vi "q2.vi"() -> ()   [LabVIEW 2015]
uses:
  <vilib>/measure/NI_MABase.lvlib
  <vilib>/Analysis/NI_AAL_SigProc.lvlib
panel:
  out "demodulated m2":dbl[](graph)=[0.19117911843553648, 0.5729591319250894, 0.5890890921294468, 1.3154738011707838, 1.3144961866221603, 1.4574064754440013, 1.42216036164409, 1.4832955134231336, 1.3040516378204707, 1.1575885486338888, 0.9909125116259979, 0.7884400558545961, 0.6256179438404917, 0.5043562747351483, 0.37651797922924957, 0.12394215236818269, 0.10483867344378245, 0.1734757640989641, 0.25167677955348666, 0.5258127619495699, 0.6110971369831356, 0.8318077101247057, 0.9128139165643081, 1.1749147514512281, 1.2134698605859797, 1.5175447967871678, 1.4551131185228479, 1.4851009517249243, 1.3185272344601384, 1.1300341180328108, 0.9606799214615833, 0.8187276271950532, 0.6530785676969499, 0.4825772132376491, 0.35900378540456035, 0.1347720355785, 0.11236091609886091, 0.17082168387920313, 0.250995683367065, 0.5240017632339953, 0.6084700995569114, 0.8350791240882549, 0.9160669423121811, 1.172037431329029, 1.2109827917652218, 1.5193252220019504, 1.4564643797442673, 1.4843749689702277, 1.3181101271518103, 1.1300576785179948, 0.9605495874632342, 0.8190225596762173, 0.6534084672462961, 0.48223614388608227, 0.3586916659088199, 0.13502194613968133, 0.11256644243782966, 0.17069219119505608, 0.2509029536063748, 0.5240390189649367, 0.6084824342437518, 0.8350964925844307, 0.9160945289287651, 1.1720012900099623, 1.2109463450464375, 1.5193581407706491, 1.4564930741484268, 1.4843539694936156, 1.3180940037118747, 1.130066624792237, 0.9605549666381606, 0.8190218097926878, 0.6534095504929038, 0.4822330218292607, 0.35868808533895324, 0.13502574918639365, 0.11256999841851738, 0.1706893219238787, 0.2509005340480438, 0.5240406167295595, 0.608483571625249, 0.8350960021102438, 0.9160943330825861, 1.1720011309259701, 1.210946060204705, 1.519358537845759, 1.4564934805140304, 1.4843535931836598, 1.318093672672127, 1.1300668708660897, 0.960555157966931, 0.8190217000510572, 0.6534094821248702, 0.48223303585579635, 0.35868807770087496, 0.13502578178268754, 0.11257003734887348, 0.17068927959896962, 0.2509004934159654, 0.5240406507580907, 0.608483600106657, 0.835095983018602, 0.9160943192608686, 1.1720011372721384, 1.2109460630840572, 1.5193585392010713, 1.4564934834001433, 1.484353588838402, 1.318093668144318, 1.1300668751438718, 0.9605551617662783, 0.8190216971708588, 0.6534094798651788, 0.4822330371897665, 0.3586880785594358, 0.13502578156357317, 0.11257003738314246, 0.170689279262532, 0.25090049299244777, 0.5240406512414064, 0.6084836005711886, 0.8350959826255947, 0.9160943189285427, 1.1720011374994639, 1.2109460632510227, 1.5193585391202487, 1.4564934833598324, 1.4843535888283999, 1.3180936681155528, 1.1300668751910647, 0.9605551618163553, 0.8190216971223002, 0.6534094798217547, 0.4822330372233053, 0.3586880785860207, 0.13502578154758946, 0.11257003737242735, 0.1706892792657163, 0.25090049299265743, 0.5240406512448724, 0.6084836005757819, 0.8350959826202083, 0.9160943189232835, 1.1720011375039954, 1.2109460632548807, 1.5193585391175606, 1.4564934833578214, 1.4843535888294235, 1.318093668116088, 1.130066875191119, 0.960555161816624, 0.8190216971217952, 0.6534094798212026, 0.4822330372238558, 0.35868807858651447, 0.1350257815472041, 0.11257003737211338, 0.17068927926590838, 0.25090049299278955, 0.5240406512448279, 0.6084836005757713, 0.835095982620178, 0.9160943189232319, 1.1720011375040587, 1.2109460632549311, 1.5193585391175148, 1.4564934833577707, 1.4843535888294634, 1.3180936681161106, 1.1300668751911107, 0.9605551618166157, 0.8190216971217973, 0.6534094798211965, 0.482233037223862, 0.3586880785865184, 0.13502578154719833, 0.1125700373721071, 0.17068927926591348, 0.2509004929927924, 0.5240406512448256, 0.6084836005757669, 0.8350959826201804, 0.9160943189232288, 1.1720011375040602, 1.2109460632549254, 1.5193585391175177, 1.456493483357764, 1.4843535888294692, 1.318093668116107, 1.130066875191115, 0.9605551618166119, 0.819021697121801, 0.6534094798211934, 0.48223303722386524, 0.35868807858651863, 0.13502578154719858, 0.11257003737210648, 0.1706892792659137, 0.25090049299279066, 0.524040651244828]
  out "demodulated m1":dbl[](graph)=[0.9667751745552262, 1.7776622875774597, 2.0989682890718457, 2.0370936358931484, 1.5938705275758451, 0.9707610204093121, 0.3798977561487974, 0.04636626851471513, 0.10574271074439387, 0.5431778625851034, 1.1662750400078337, 1.75714886772281, 2.10065564741628, 2.036961451408783, 1.5938803423381982, 0.9707603267524426, 0.37989780244737176, 0.04636626932203434, 0.10574271096034764, 0.5431778625782561, 1.16627504000793, 1.7571488677228333, 2.100655647416275, 2.0369614514087817, 1.5938803423381962, 0.9707603267524398, 0.37989780244737087, 0.04636626932203441, 0.1057427109603482, 0.5431778625782558, 1.1662750400079291, 1.7571488677228326, 2.100655647416274, 2.0369614514087813, 1.5938803423381949, 0.9707603267524393, 0.3798978024473701, 0.04636626932203515, 0.10574271096034787, 0.5431778625782563, 1.166275040007929, 1.7571488677228333, 2.1006556474162728, 2.0369614514087804, 1.5938803423381924, 0.9707603267524383, 0.379897802447369, 0.04636626932203517, 0.10574271096034844, 0.5431778625782572, 1.1662750400079296, 1.7571488677228326, 2.100655647416272, 2.0369614514087777, 1.5938803423381926, 0.9707603267524362, 0.37989780244736876, 0.04636626932203555, 0.10574271096034833, 0.5431778625782572, 1.1662750400079311, 1.757148867722834, 2.100655647416276, 2.0369614514087746, 1.593880342338191, 0.9707603267524332, 0.37989780244736615, 0.04636626932203414, 0.10574271096035096, 0.5431778625782598, 1.1662750400079338, 1.7571488677228337, 2.100655647416276, 2.036961451408773, 1.5938803423381895, 0.9707603267524307, 0.37989780244736493, 0.046366269322034026, 0.10574271096035118, 0.5431778625782602, 1.1662750400079345, 1.757148867722833, 2.1006556474162736, 2.03696145140877, 1.5938803423381864, 0.9707603267524283, 0.3798978024473641, 0.04636626932203422, 0.10574271096035187, 0.5431778625782613, 1.166275040007934, 1.7571488677228322, 2.100655647416272, 2.036961451408767, 1.5938803423381838, 0.9707603267524264, 0.37989780244736293, 0.046366269322034366, 0.10574271096035236, 0.5431778625782615]
  out "input m2":waveform(dbl)(graph)={"t0"=timestamp(0 s since 1904-01-01), "dt"=0.002, "Y"=array[500 elements]}
  out "input m1":waveform(dbl)(graph)={"t0"=timestamp(0 s since 1904-01-01), "dt"=0.002, "Y"=array[500 elements]}
  in  "sampling info":cluster{"Fs":dbl, "#s":dbl}={"Fs"=500.0, "#s"=500.0} {"Fs" format="%.2p"}
  in  "signal type":T1(ring)
  in  "amplitude 2":dbl=1.0 format="%0.2p"
  in  "fc2":dbl=200.0 format="%0.2p"
  in  "sampling info 2":cluster{"Fs":dbl, "#s":dbl}={"Fs"=500.0, "#s"=500.0} {"Fs" format="%.2p"}
  in  "signal type":T1(ring)=enum."Triangle Wave"
  in  "amplitude 2":dbl=1.0 format="%0.2p"
  in  "fm2":dbl=10.0 format="%0.2p"
  in  "sampling info":cluster{"Fs":dbl, "#s":dbl}={"Fs"=500.0, "#s"=500.0} {"Fs" format="%.2p"}
  in  "signal type":T1(ring)
  in  "amplitude 1":dbl=1.0 format="%0.2p"
  in  "fc1":dbl=100.0 format="%0.2p"
  in  "sampling info":cluster{"Fs":dbl, "#s":dbl}={"Fs"=500.0, "#s"=500.0} {"Fs" format="%.2p"}
  in  "signal type":T1(ring)
  in  "amplitude 1":dbl=1.0 format="%0.2p"
  in  "fm1":dbl=10.0 format="%0.2p"
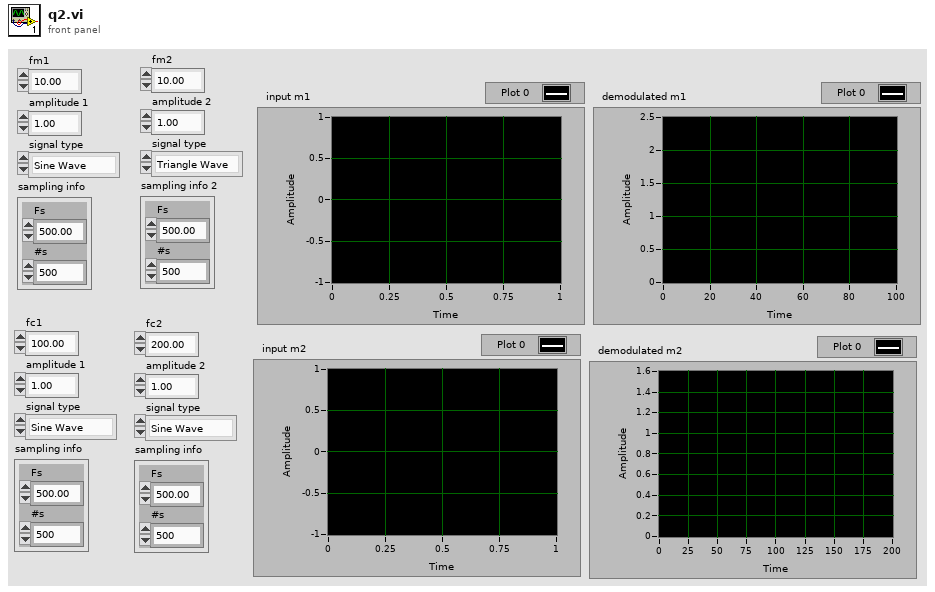
[diagram p1: front panel]
types:
  T1 = enum16{"Sine Wave", "Triangle Wave", "Square Wave", "Sawtooth Wave"}
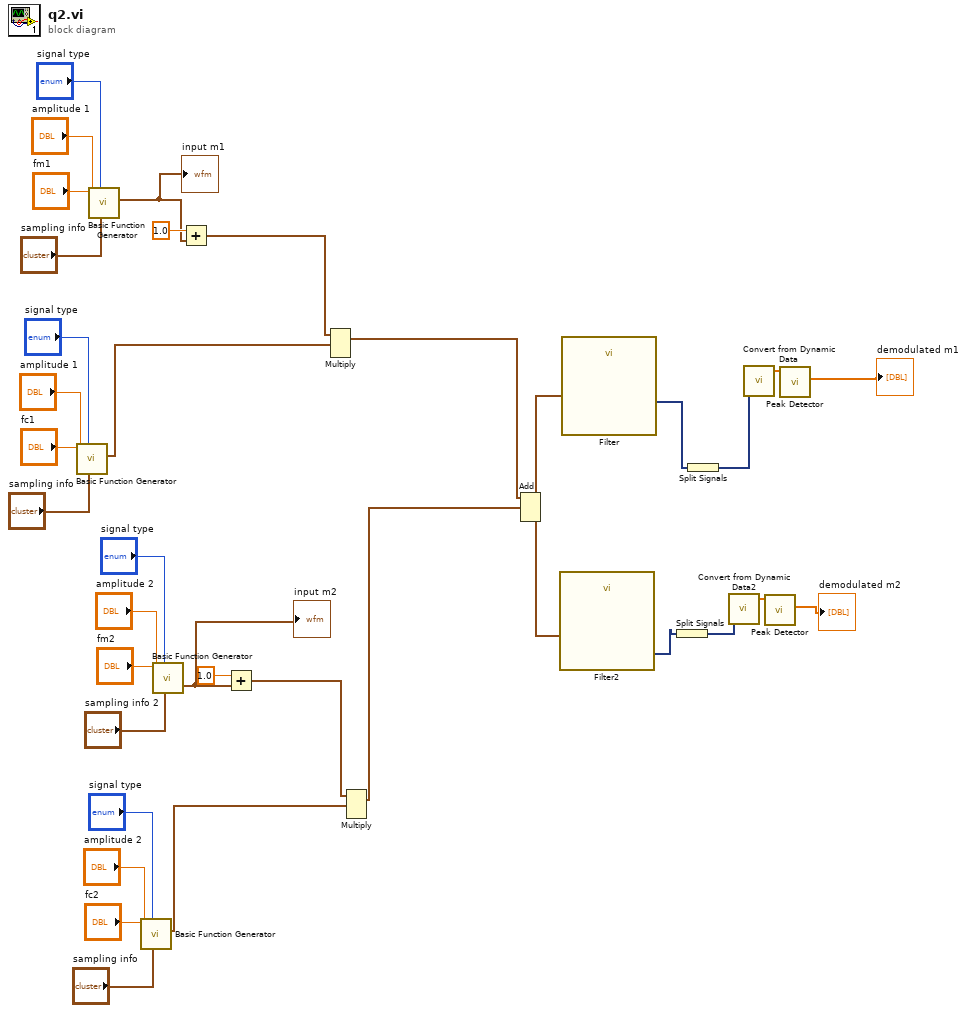
[diagram p0: block diagram]
diagram:
  n1 = call <vilib>:"Basic Function Generator.vi"("sampling info"="sampling info", "signal type"="signal type", "amplitude"="amplitude 1", "frequency"="fc1") -> ("signal out"=w17:waveform(dbl))  [unwired: 5 in, 2 out]
  n2 = call <vilib>:"Basic Function Generator.vi"("sampling info"="sampling info", "signal type"="signal type", "amplitude"="amplitude 1", "frequency"="fm1") -> ("signal out"=w1:waveform(dbl))  [unwired: 5 in, 2 out]
  "input m1" <- w1
  n3 = call <vilib>:"Basic Function Generator.vi"("sampling info"="sampling info", "signal type"="signal type", "amplitude"="amplitude 2", "frequency"="fc2") -> ("signal out"=w15:waveform(dbl))  [unwired: 5 in, 2 out]
  n4 = call <vilib>:"Basic Function Generator.vi"("sampling info"="sampling info 2", "signal type"="signal type", "amplitude"="amplitude 2", "frequency"="fm2") -> ("signal out"=w2:waveform(dbl))  [unwired: 5 in, 2 out]
  "input m2" <- w2
  n5 = Add(x=1.0, y=w1) -> (x+y=w5:waveform(dbl))
  n6 = Add(x=1.0, y=w2) -> (x+y=w16:waveform(dbl))
  n7 = Multiply(1:w17, 2:w5) -> (0:w3:waveform(dbl))  [unwired: 1 in, 1 out]
  n8 = Multiply(1:w15, 2:w16) -> (0:w4:waveform(dbl))  [unwired: 1 in, 1 out]
  n9 = Add(1:w4, 2:w3) -> (0:w14:waveform(dbl))  [unwired: 1 in, 1 out]
  n10 = call "Filter2"("Signal"=w14) -> ("Filtered Signal"=w10:dynamicdata)  [unwired: 9 in, 1 out]
  n11 = call "Filter"("Signal"=w14) -> ("Filtered Signal"=w13:dynamicdata)  [unwired: 9 in, 1 out]
  n12 = Split Signals(w10) -> (w9:dynamicdata)  [unwired: 1 in]
  n13 = Split Signals(w13) -> (w12:dynamicdata)  [unwired: 1 in]
  n14 = call "Convert from Dynamic Data2"("Dynamic Data Type"=w9) -> ("Array"=w8:dbl[])  [unwired: 3 in]
  n15 = call "Convert from Dynamic Data"("Dynamic Data Type"=w12) -> ("Array"=w11:dbl[])  [unwired: 3 in]
  n16 = call <vilib>:"Peak Detector.vi"("X"=w8) -> ("Amplitudes"=→"demodulated m2":dbl[])  [unwired: 6 in, 4 out]
  n17 = call <vilib>:"Peak Detector.vi"("X"=w11) -> ("Amplitudes"=→"demodulated m1":dbl[])  [unwired: 6 in, 4 out]
